vi "Get Events.vi"(11 "Sensor Charm View in":refnum<class "Sensor Charm View.lvclass">) -> (2 "Events":T1, 3 "Sensor Charm View out":refnum<class "Sensor Charm View.lvclass">)   [LabVIEW 2013, in "Sensor Charm View.lvlib" / "Sensor Charm View.lvclass"]
uses:
  Sensor Charm View.lvclass
  Typedef/Events.ctl
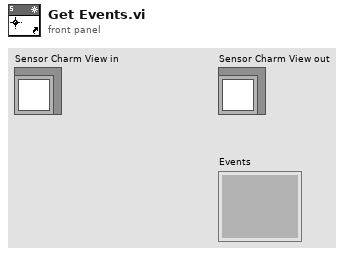
[diagram p1: front panel]
types:
  T1 = typedef "Sensor Charm View.lvlib/Sensor Charm View.lvclass/Events.ctl" = cluster{}
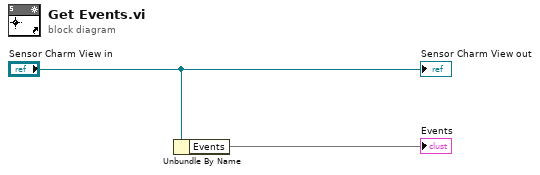
[diagram p0: block diagram]
diagram:
  n1 = Unbundle By Name("Sensor Charm View in") -> ("Events"=→"Events")
  "Sensor Charm View out" <- "Sensor Charm View in"
